vi "Teste de processamento de dados.vi"() -> ()   [LabVIEW 2016]
uses:
  <vilib>/addons/_JKI Toolkits/Caraya/classes/Assert/Assert.lvclass
  <vilib>/addons/_JKI Toolkits/Caraya/classes/Test/Test.lvclass
panel:
  out "error out":errorcluster
  in  "error in (no error)":errorcluster
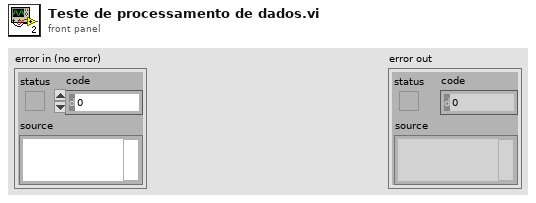
[diagram p1: front panel]
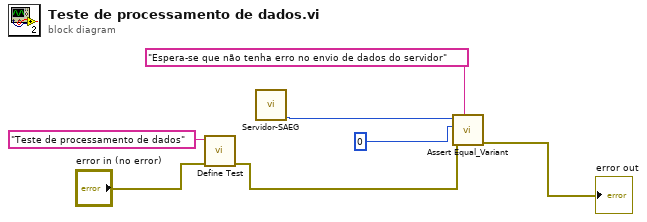
[diagram p0: block diagram]
diagram:
  n1 = call <vilib>:"Define Test.vi"("error in (no error)"="error in (no error)", "Label (VI Title)"="Teste de processamento de dados") -> ("error out"=w4:errorcluster)  [unwired: 9 in]
  n2 = call "Servidor-SAEG.vi"() -> ("error"=w7:i32)  [unwired: 10 in, 1 out]
  n3 = call <vilib>:"Assert Equal_Variant.vi"("Label"="Espera-se que não tenha erro no envio de dados do servidor", "error in (no error)"=w4, "Y"=0, "X"=w7) -> ("error out"=→"error out":errorcluster)  [unwired: 7 in]
